vi "DAQ_SV Gen Initialize.vi"(0 "Physical Channels":tag, 7 "Global Channels":refnum<k21>, 11 "error in":errorcluster) -> (4 "DAQmx Task Out":refnum<k21>, 15 "error out":errorcluster)   [LabVIEW 2021, in "DAQ_Signal Voltage Generation.lvlib"]
doc: "Initialize analog output channels and obtains a DAQmx task\n\nProvide either Physical channel or Global Channel\nIf both physical and Global channels are provided, Global Channels will take precedences"
uses:
  DAQ_Signal Voltage Generation.lvlib
  <vilib>/DAQmx/create/channels.llb/DAQmx Create Channel (AO-Voltage-Basic).vi
panel:
  # "Inputs"
  # "Outputs"
  # "Overview:\nThis VI initializes an analog output session and provides the DAQmx Task Out\n\nHardware Requirement: A compatible PXI, PCIe, USB, cDAQ or Testscale device\n\nSoftware Requirement: NI DAQmx 2022 Q4 or later\n\nInstructions:\n1. Enter physical channel in which Signal voltage generation has to be done in Physical Channels control. (Or) Enter Global channels to use it instead of initiating a new task. User must configure only one input. If both are mentioned, Global Channels will take precedence.\n3. Get the Signal voltage generation task from DAQmx Task Out\n\nNote: User can use the DAQmx Task on other VIs to configure and initiate signal voltage generation."
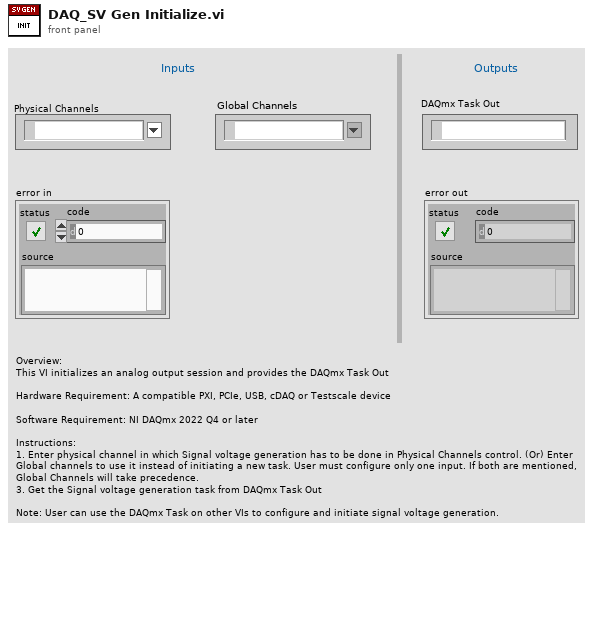
[diagram p1: front panel]
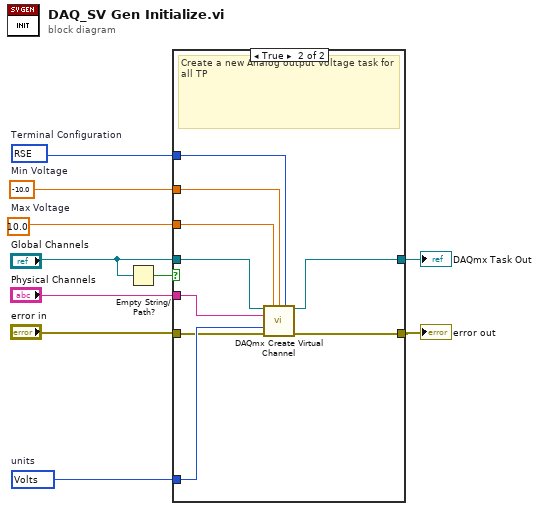
[diagram p0: block diagram]
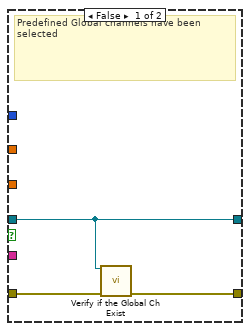
[diagram p2: hidden frame]
diagram:
  w10 = 10083 items=["RSE"=10083, "NRSE"=10078, "Differential"=10106]  # Terminal Configuration
  w9 = -10.0  # Min Voltage
  w8 = 10.0  # Max Voltage
  w6 = 10348 items=["Volts"=10348, "From Custom Scale"=10065]  # units
  n1 = Empty String/Path?(string/path="Global Channels") -> (empty?=w1:bool)
  n2 = case shown="True" w1 {
    tunnel: "Physical Channels" -> [_ w14]
    tunnel: w10 -> [_ w22]
    tunnel: w9 -> [_ w21]
    tunnel: w8 -> [_ w20]
    tunnel: "Global Channels" -> [w11 w19]
    tunnel: [w11 w18] -> w5
    tunnel: "error in" -> [w13 w15]
    tunnel: [w12 w17] -> w4
    tunnel: w6 -> [_ w16]
    frame False {
      # "Predefined Global channels have been selected"
      n3 = call "Verify if the Global Ch Exist.vi"("Global Channels"=w11, "error in (no error)"=w13) -> ("error out"=w12:errorcluster)  [unwired: 13 in]
    }
    frame True {
      # "Create a new Analog output Voltage task for all TP"
      n4 = call-poly <vilib>:"DAQmx Create Virtual Channel.vi"("task in"=w19, "maximum value"=w20, "minimum value"=w21, "output terminal configuration"=w22, "physical channels"=w14, "units"=w16, "error in"=w15) -> ("task out"=w18:refnum<k21>, "error out"=w17:errorcluster)  [unwired: 7 in]
    }
  }
  "DAQmx Task Out" <- w5
  "error out" <- w4
